vi "UpdateFrontPanel.vi"(8 "error in":errorcluster, 10 "Cluster":T1, 11 "Waveform Specification in":T2) -> (0 "error out":errorcluster, 3 "Waveform Specification out":T2)   [LabVIEW 2017, in "WaveformGenerator.lvlib"]
uses:
  WaveformGenerator.lvlib
  WaveformSpecs.ctl
  WaveformGeneratorInterfaceRef.ctl
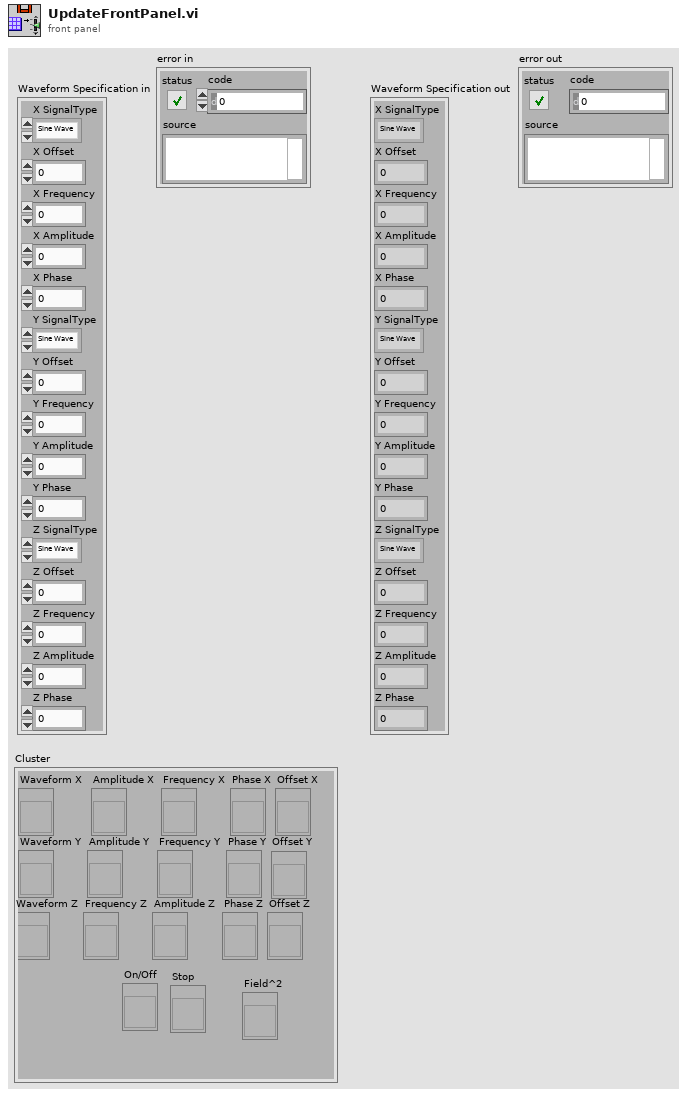
[diagram p1: front panel]
types:
  T1 = typedef "WaveformGenerator.lvlib/WaveformGeneratorInterfaceRef.ctl" = cluster{"Waveform X":refnum<vi>, "Waveform Y":refnum<vi>, "Waveform Z":refnum<vi>, "Amplitude X":refnum<vi>, "Amplitude Y":refnum<vi>, "Amplitude Z":refnum<vi>, "Frequency X":refnum<vi>, "Frequency Y":refnum<vi>, "Frequency Z":refnum<vi>, "Phase X":refnum<vi>, "Phase Y":refnum<vi>, "Phase Z":refnum<vi>, "Offset X":refnum<vi>, "Offset Y":refnum<vi>, "Offset Z":refnum<vi>, "Stop":refnum<vi>, "On/Off":refnum<vi>, "Field^2":refnum<vi>}
  T2 = typedef "WaveformGenerator.lvlib/WaveformSpecs.ctl" = cluster{"X SignalType":enum16{"Sine Wave", "Triangle Wave", "Square Wave", "Sawtooth Wave"}, "X Offset":dbl, "X Frequency":dbl, "X Amplitude":dbl, "X Phase":dbl, "Y SignalType":enum16{"Sine Wave", "Triangle Wave", "Square Wave", "Sawtooth Wave"}, "Y Offset":dbl, "Y Frequency":dbl, "Y Amplitude":dbl, "Y Phase":dbl, "Z SignalType":enum16{"Sine Wave", "Triangle Wave", "Square Wave", "Sawtooth Wave"}, "Z Offset":dbl, "Z Frequency":dbl, "Z Amplitude":dbl, "Z Phase":dbl}
  T3 = enum16{"Sine Wave", "Triangle Wave", "Square Wave", "Sawtooth Wave"}
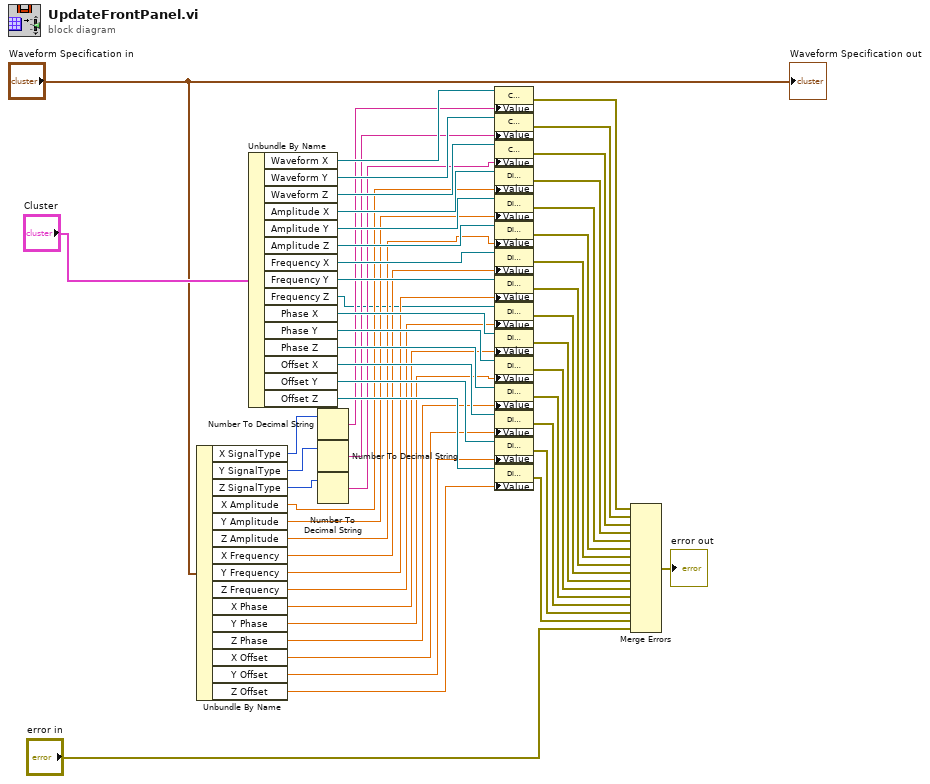
[diagram p0: block diagram]
diagram:
  n1 = Unbundle By Name("Waveform Specification in") -> ("X SignalType"=w19:T3, "Y SignalType"=w18:T3, "Z SignalType"=w17:T3, "X Amplitude"=w13:dbl, "Y Amplitude"=w12:dbl, "Z Amplitude"=w11:dbl, "X Frequency"=w10:dbl, "Y Frequency"=w9:dbl, "Z Frequency"=w7:dbl, "X Phase"=w6:dbl, "Y Phase"=w5:dbl, "Z Phase"=w4:dbl, "X Offset"=w3:dbl, "Y Offset"=w2:dbl, "Z Offset"=w1:dbl)
  n2 = Unbundle By Name("Cluster") -> ("Waveform X"=w39:refnum<vi>, "Waveform Y"=w40:refnum<vi>, "Waveform Z"=w41:refnum<vi>, "Amplitude X"=w42:refnum<vi>, "Amplitude Y"=w43:refnum<vi>, "Amplitude Z"=w44:refnum<vi>, "Frequency X"=w45:refnum<vi>, "Frequency Y"=w46:refnum<vi>, "Frequency Z"=w8:refnum<vi>, "Phase X"=w47:refnum<vi>, "Phase Y"=w48:refnum<vi>, "Phase Z"=w52:refnum<vi>, "Offset X"=w49:refnum<vi>, "Offset Y"=w50:refnum<vi>, "Offset Z"=w51:refnum<vi>)
  n3 = Number To Decimal String(number=w19) -> (decimal integer string=w16:string)  [unwired: 1 in]
  n4 = Number To Decimal String(number=w18) -> (decimal integer string=w15:string)  [unwired: 1 in]
  n5 = Number To Decimal String(number=w17) -> (decimal integer string=w14:string)  [unwired: 1 in]
  n6 = property class="CmbBox"(reference=w39, "Value"=w16) -> (error out=w23:errorcluster)  [unwired: 1 in, 1 out]
  n7 = property class="CmbBox"(reference=w40, "Value"=w15) -> (error out=w24:errorcluster)  [unwired: 1 in, 1 out]
  n8 = property class="CmbBox"(reference=w41, "Value"=w14) -> (error out=w25:errorcluster)  [unwired: 1 in, 1 out]
  n9 = property class="DigNum (strict)"(reference=w42, "Value"=w13) -> (error out=w26:errorcluster)  [unwired: 1 in, 1 out]
  n10 = property class="DigNum (strict)"(reference=w43, "Value"=w12) -> (error out=w27:errorcluster)  [unwired: 1 in, 1 out]
  n11 = property class="DigNum (strict)"(reference=w44, "Value"=w11) -> (error out=w28:errorcluster)  [unwired: 1 in, 1 out]
  n12 = property class="DigNum (strict)"(reference=w45, "Value"=w10) -> (error out=w29:errorcluster)  [unwired: 1 in, 1 out]
  n13 = property class="DigNum (strict)"(reference=w46, "Value"=w9) -> (error out=w30:errorcluster)  [unwired: 1 in, 1 out]
  n14 = property class="DigNum (strict)"(reference=w8, "Value"=w7) -> (error out=w31:errorcluster)  [unwired: 1 in, 1 out]
  n15 = property class="DigNum (strict)"(reference=w47, "Value"=w6) -> (error out=w32:errorcluster)  [unwired: 1 in, 1 out]
  n16 = property class="DigNum (strict)"(reference=w48, "Value"=w5) -> (error out=w33:errorcluster)  [unwired: 1 in, 1 out]
  n17 = property class="DigNum (strict)"(reference=w52, "Value"=w4) -> (error out=w34:errorcluster)  [unwired: 1 in, 1 out]
  n18 = property class="DigNum (strict)"(reference=w49, "Value"=w3) -> (error out=w35:errorcluster)  [unwired: 1 in, 1 out]
  n19 = property class="DigNum (strict)"(reference=w50, "Value"=w2) -> (error out=w36:errorcluster)  [unwired: 1 in, 1 out]
  n20 = property class="DigNum (strict)"(reference=w51, "Value"=w1) -> (error out=w37:errorcluster)  [unwired: 1 in, 1 out]
  n21 = Merge Errors(w23, w24, w25, w26, w27, w28, w29, w30, w31, w32, w33, w34, w35, w36, w37, "error in") -> (→"error out":errorcluster)
  "Waveform Specification out" <- "Waveform Specification in"
